vi "ReadContent.vi"(8 "error in (no error)":errorcluster, 11 "object in":refnum<class "shutdown_request Message.lvclass">) -> (0 "error out":errorcluster, 2 "content":string, 3 "object out":refnum<class "shutdown_request Message.lvclass">)   [LabVIEW 2018]
uses:
  744fdd79-a514-42eb-8e88-aec33424e066.vi
  shutdown_request Message/shutdown_request Message.lvclass
  C:/Users/gavin/Documents/LabVIEW Data/LabVIEW-Bits/Connectivity/Jupyter Client/Base Classes/Request Message/Request Message.lvclass
  C:/Users/gavin/Documents/LabVIEW Data/LabVIEW-Bits/Connectivity/Jupyter Client/Base Classes/Message Class/Message Class.lvclass
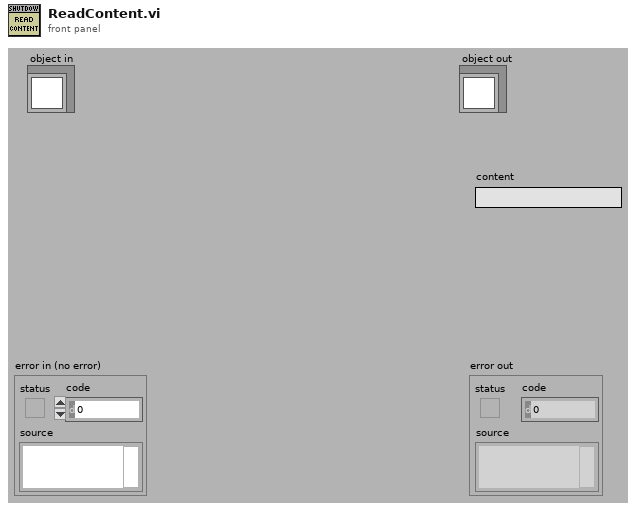
[diagram p1: front panel]
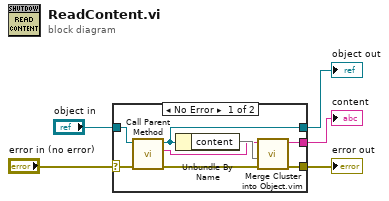
[diagram p0: block diagram]
diagram:
  n1 = case shown="No Error" "error in (no error)" {
    selector: "error in (no error)" -> [w7 w15]
    tunnel: [w6 w15] -> w4
    tunnel: [w11 w14] -> w2
    tunnel: "object in" -> [w13 w14]
    tunnel: [w8 _] -> w1
    frame No Error {
      n2 = call-parent "Call Parent Method"("error in (no error)"=w7, "object in"=w13) -> ("error out"=w9:errorcluster, "content"=w10:string, "object out"=w11:refnum<class "shutdown_request Message.lvclass">)  [unwired: 7 in]
      n3 = Unbundle By Name(w11) -> ("content"=w12)
      n4 = call "Merge Cluster into Object.vim"("error in (no error)"=w9, "Any Cluster"=w12, "JSON"=w10) -> ("error out"=w6:errorcluster, "<JSON>"=w8:string)  [unwired: 6 in]
    }
    frame Error {
    }
  }
  "error out" <- w4
  "object out" <- w2
  "content" <- w1
